vi "Drive Get.vi"(6 "error in (no error)":errorcluster, 8 "Show off spin":bool, 9 "Slow Drive":bool, 10 "Y - Axis":dbl, 11 "X - Axis":dbl) -> (0 "error out":errorcluster)   [LabVIEW 2013]
uses:
  Drive Global.vi
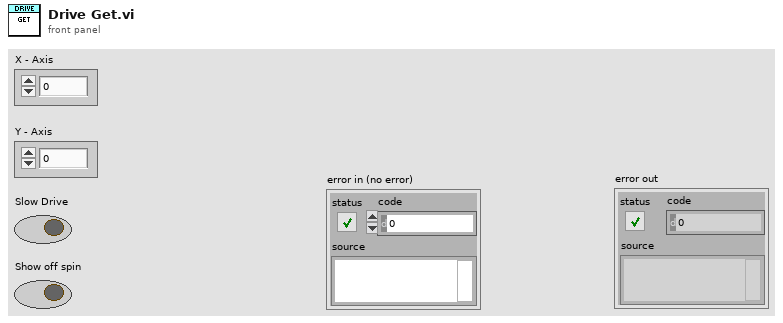
[diagram p1: front panel]
types:
  T1 = cluster{"X Axis":dbl, "Y Axis":dbl, "Slow Drive":bool, "Show Off Spin":bool, "Hands Off":bool, "Right Gear Distance":dbl, "Left Gear Distance ":dbl, "Right Gear RPM":dbl, "Left Gear RPM":dbl}
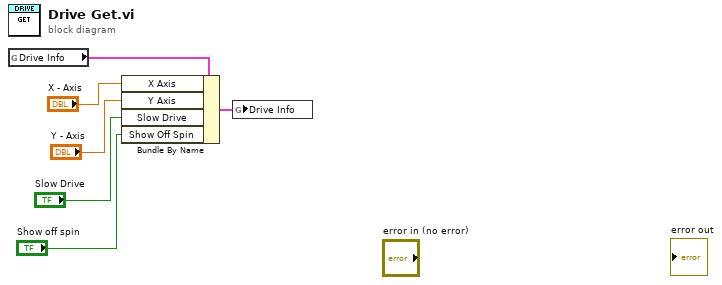
[diagram p0: block diagram]
diagram:
  n1 = global read "Drive Global.vi" "Drive Info"() -> (w5:T1)
  n2 = Bundle By Name(cluster=w5, "X Axis"="X - Axis", "Y Axis"="Y - Axis", "Slow Drive"="Slow Drive", "Show Off Spin"="Show off spin") -> (w6:T1)
  n3 = global write "Drive Global.vi" "Drive Info"(w6) -> ()
